vi "VariantToProperties.vi"(8 "error in (no error)":errorcluster, 11 "ChromaPowerSupply in":refnum<class "ChromaPowerSupply.lvclass">) -> (0 "error out":errorcluster, 1 "Measurements":T2, 2 "Device Settings":T1 caption="Device(s)Settings", 3 "ChromaPowerSupply out":refnum<class "ChromaPowerSupply.lvclass">, 4 "Measurement Refresh Time (ms)":u32)   [LabVIEW 2018, in "AcPwrPlugins.lvlib" / "ChromaPowerSupply.lvclass"]
uses:
  ChromaPowerSupply.lvclass
  C:/Users/Public/Projects/ICDAS/NistPluggableModules/AcPwr/AcPwrPlugins/AcPwrBaseClass/AcPwrBase.lvclass
  TypeDefs/Measurements.ctl
  TypeDefs/Device(s)Settings.ctl
  AcPwrBaseClass/AcPwrBase.lvclass/AcPwrBase.ctl
  AcPwrBaseClass/Accessors/Read BaseConfig.vi
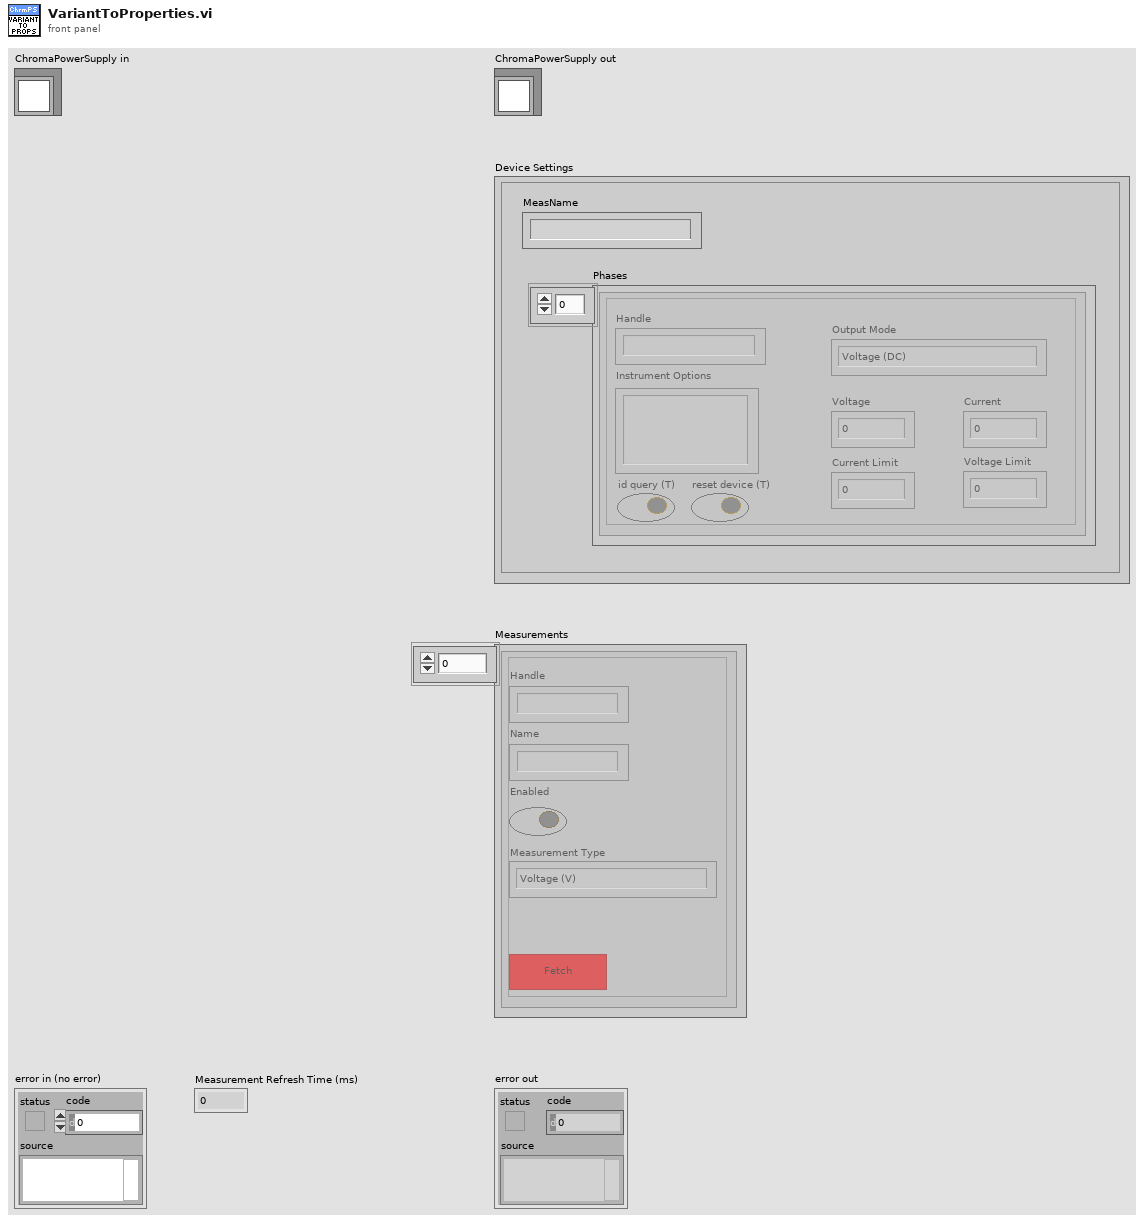
[diagram p1: front panel]
types:
  T1 = typedef "AcPwrPlugins.lvlib/ChromaPowerSupply.lvclass/Device(s)Settings.ctl" = cluster{"Phases":cluster{"Handle":string, "Instrument Options":string, "id query (T)":bool, "reset device (T)":bool, "Timing":cluster{"TimingOn":enum16{""}, "Hours":u32, "Minutes":u32, "Seconds":dbl, "CutoffVoltage":dbl}, "Connected":bool, "Output Mode":enum16{"Voltage (DC)", "Current (DC)"}, "Voltage":dbl, "Current":dbl, "Voltage Limit":dbl, "Current Limit":dbl}[], "MeasName":string}
  T2 = typedef "AcPwrPlugins.lvlib/ChromaPowerSupply.lvclass/Measurements.ctl" = cluster{"Handle":string, "Name":string, "Enabled":bool, "Measurement Value":dbl, "btnMeasFetch":bool, "ProtectionStatusString":string, "Measurement Type":enum16{"Voltage (V)", "Current (A)", "Power (W)"}}[]
  T3 = typedef "AcPwrPlugins.lvlib/AcPwrBase.lvclass/BaseConfig.ctl" = cluster{"Frequency":dbl, "FrequencyRange":dbl[], "Phases":T4[], "Name":string, "PluginConfigVariant":variant, "PluginMeasVariant":variant}
  T4 = typedef "AcPwrPlugins.lvlib/AcPwrBase.lvclass/Phase.ctl" = cluster{"Name":string, "Enabled":bool, "VoltageLevel":dbl, "Handle":string, "VoltageRange":dbl[], "Connected":bool, "CurrentLimit":dbl, "Waveform":string}
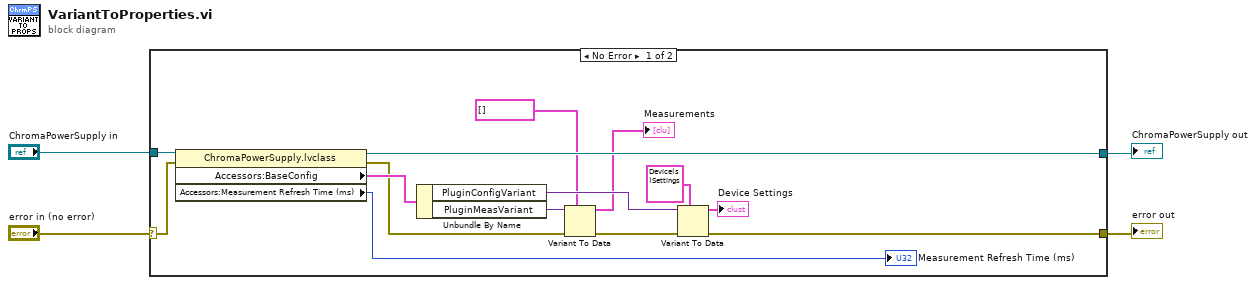
[diagram p0: block diagram]
diagram:
  n1 = case shown="No Error" "error in (no error)" {
    selector: "error in (no error)" -> [w16 w20]
    tunnel: [w18 w20] -> w1
    tunnel: "ChromaPowerSupply in" -> [w17 w19]
    tunnel: [w15 w19] -> w2
    frame No Error {
      n2 = property class="ChromaPowerSupply.lvclass"(reference=w17, error in=w16) -> (reference out=w15:refnum<class "ChromaPowerSupply.lvclass">, error out=w13:errorcluster, "Accessors:BaseConfig"=w14:T3, "Accessors:Measurement Refresh Time (ms)"=→"Measurement Refresh Time (ms)":u32)
      n3 = Unbundle By Name(w14) -> ("PluginConfigVariant"=w10:variant, "PluginMeasVariant"=w12:variant)
      n4 = Variant To Data(error in=w13, type=T2 [] ("Measurements"), Variant=w12) -> (data=→"Measurements":T2, error out=w11:errorcluster)
      n5 = Variant To Data(error in=w11, type=T1 {"Phases"=[{"Handle"="", "Instrument Options"="", "id query (T)"=TRUE, "reset device (T)"=TRUE, "Timing"={"TimingOn"=enum."", "Hours"=0, "Minutes"=0, "Seconds"=0.0, "CutoffVoltage"=0.0}, "Connected"=FALSE, "Output Mode"=enum."Voltage (DC)", "Voltage"=0.0, "Current"=0.0, "Voltage Limit"=0.0, "Current Limit"=0.0}], "MeasName"=""} ("Device(s)Settings"), Variant=w10) -> (data=→"Device Settings":T1, error out=w18:errorcluster)
    }
    frame Error {
    }
  }
  "error out" <- w1
  "ChromaPowerSupply out" <- w2
